vi "Get String Value.vi"(6 "Default Value":string, 8 "error in (no error)":errorcluster, 10 "Name":string, 11 "Test Recipe in":refnum<class "Test Recipe.lvclass">) -> (0 "error out":errorcluster, 1 "found?":bool, 2 "Value":string, 3 "Test Recipe out":refnum<class "Test Recipe.lvclass">)   [LabVIEW 2015, in "Test Recipe.lvlib" / "Test Recipe.lvclass"]
uses:
  Test Recipe.lvclass
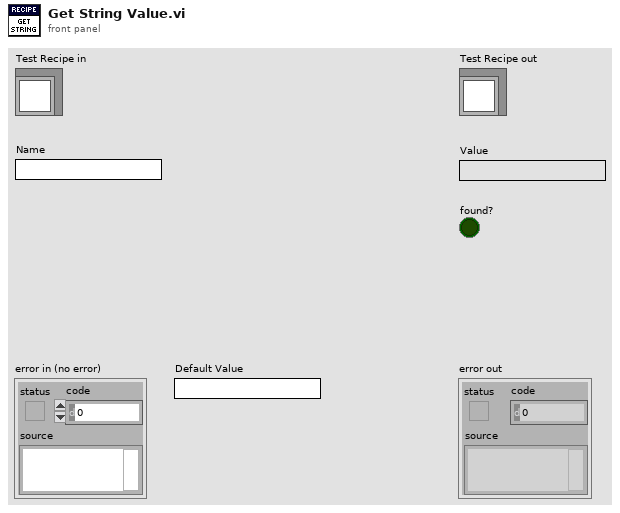
[diagram p1: front panel]
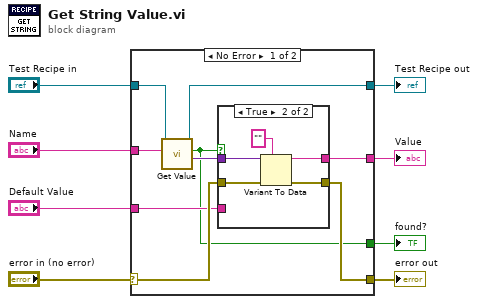
[diagram p0: block diagram]
diagram:
  n1 = case shown="No Error" "error in (no error)" {
    selector: "error in (no error)" -> [w12 w26]
    tunnel: [w11 w26] -> w7
    tunnel: [w16 w25] -> w5
    tunnel: "Test Recipe in" -> [w17 w25]
    tunnel: "Name" -> [w15 _]
    tunnel: [w13 _] -> w3
    tunnel: "Default Value" -> [w10 _]
    tunnel: [w9 _] -> w1
    frame No Error {
      n2 = call-dynamic "Get Value.vi"("Key"=w15, "Registry in"=w17) -> ("Value"=w14:variant, "found?"=w9:bool, "Registry out"=w16:refnum<class "Test Recipe.lvclass">)  [unwired: 6 in, 1 out]
      n3 = case shown="True" w9 {
        tunnel: w14 -> [_ w24]
        tunnel: [w18 w23] -> w13
        tunnel: w12 -> [w19 w22]
        tunnel: [w19 w21] -> w11
        tunnel: w10 -> [w18 _]
        frame False {
        }
        frame True {
          n4 = Variant To Data(error in=w22, type="", Variant=w24) -> (data=w23:string, error out=w21:errorcluster)
        }
      }
    }
    frame Error {
    }
  }
  "error out" <- w7
  "Test Recipe out" <- w5
  "Value" <- w3
  "found?" <- w1
